vi "USB - Discover DAQ Devices on USB to Serial Ports.vi"(8 "error in":errorcluster) -> (0 "error out":errorcluster, 2 "Number of Devices Found":i32, 3 "List of DAQiFi COM Ports":string[](array[string]))   [LabVIEW 2021]
uses:
  <vilib>/Instr/_visa.llb/VISA Find Search Mode.ctl
  <vilib>/Instr/_visa.llb/VISA Configure Serial Port (Instr).vi
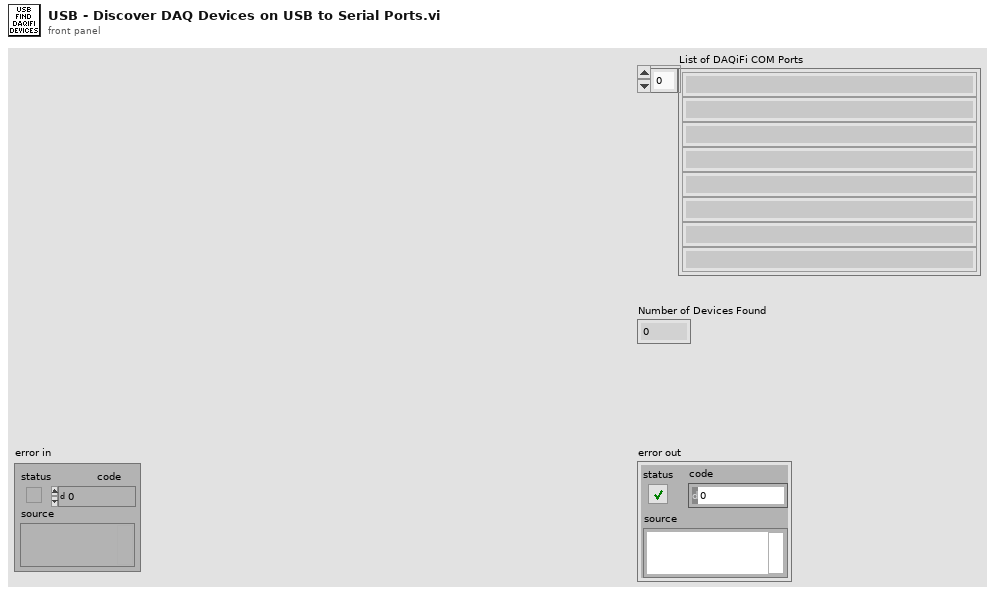
[diagram p1: front panel]
types:
  T1 = typedef "VISA Find Search Mode.ctl" = u32
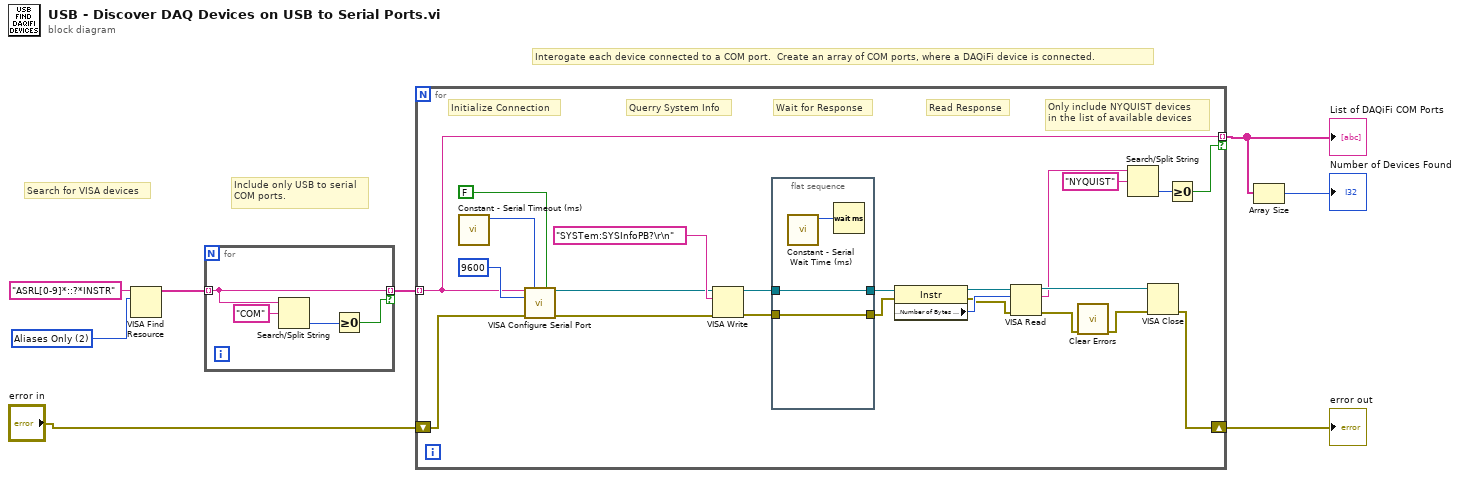
[diagram p0: block diagram]
diagram:
  w7 = T1 2 items=["Canonical Names Only"=0, "Aliases Only"=2, "Include Matching Aliases"=3, "Include All Aliases"=4] ("Search Mode")
  # "Interogate each device connected to a COM port.  Create an array of COM ports, where a DAQiFi device is connected."
  # "Include only USB to serial\nCOM ports."
  # "Search for VISA devices"
  n1 = VISA Find Resource(10:w7, 11:"ASRL[0-9]*::?*INSTR" ("expression (\"?*\")")) -> (3:w6:string[])  [unwired: 1 in, 2 out]
  n2 = for {
    tunnel: w6 -> [w12] mode=indexing
    tunnel: [w12] -> w5 mode=indexing if=w9
    n3 = Search/Split String(string=w12, search string/char (-)="COM") -> (offset of match=w10:i32)  [unwired: 1 in, 2 out]
    n4 = Greater Or Equal To 0?(x=w10) -> (x >= 0?=w9:bool)
  }
  n5 = for {
    tunnel: w5 -> [w15] mode=indexing
    tunnel: [w15] -> w2 mode=indexing if=w16
    shift-right: [w13] -> w3
    shift-left: "error in" -> [w14]
    # "Only include NYQUIST devices\nin the list of available devices"
    # "Read Response"
    # "Wait for Response"
    # "Querry System Info"
    # "Initialize Connection"
    n6 = call "Constant - Serial Timeout (ms).vi"() -> ("timeout (ms)"=w22:i32)  [unwired: 11 in]
    n7 = call-poly "VISA Configure Serial Port"("VISA resource name"=w15, "timeout (10sec)"=w22, "Enable Termination\nChar (T)"=FALSE ("Enable Termination\nChar (T)"), "baud rate (9600)"=u32 9600, "error in (no error)"=w14) -> ("VISA resource name out"=w28:refnum<visa-resource-name>, "error out"=w29:errorcluster)  [unwired: 9 in]
    n8 = VISA Write(VISA resource name=w28, write buffer="SYSTem:SYSInfoPB?\r\n", error in (no error)=w29) -> (VISA resource name out=w27:refnum<visa-resource-name>, error out=w25:errorcluster)  [unwired: 1 out]
    n9 = flat-sequence {
      tunnel: [w38] -> w26
      tunnel: w27 -> [w38]
      tunnel: w25 -> [w37]
      tunnel: [w37] -> w24
      frame #0 {
        n10 = call "Constant - Serial Wait Time (ms).vi"() -> ("milliseconds to wait"=w36:u32)  [unwired: 11 in]
        n11 = Wait (ms)(milliseconds to wait=w36) -> ()  [unwired: 1 out]
      }
    }
    n12 = property class="Instr"(reference=w26, error in=w24) -> (reference out=w31:refnum<visa-resource-name>, error out=w32:errorcluster, "Serial Settings:Number of Bytes at Serial Port"=w33:u32)
    n13 = VISA Read(VISA resource name=w31, byte count=w33, error in (no error)=w32) -> (VISA resource name out=w30:refnum<visa-resource-name>, read buffer=w17:string, error out=w21:errorcluster)  [unwired: 1 out]
    n14 = call <vilib>:"Clear Errors.vi"("error in (no error)"=w21) -> ("error out"=w20:errorcluster)  [unwired: 5 in, 1 out]
    n15 = Search/Split String(string=w17, search string/char (-)="NYQUIST") -> (offset of match=w18:i32)  [unwired: 1 in, 2 out]
    n16 = VISA Close(VISA resource name=w30, error in (no error)=w20) -> (error out=w13:errorcluster)
    n17 = Greater Or Equal To 0?(x=w18) -> (x >= 0?=w16:bool)
  }
  "List of DAQiFi COM Ports" <- w2
  "error out" <- w3
  n18 = Array Size(array=w2) -> (size(s)=→"Number of Devices Found":i32)
